vi "Read CellPart.vi"(8 "error in (no error)":errorcluster, 11 "TreeDoubleClickMsg in":refnum<class "TreeDoubleClickMsg.lvclass">) -> (0 "error out":errorcluster, 2 "CellPart":T1(ring), 3 "TreeDoubleClickMsg out":refnum<class "TreeDoubleClickMsg.lvclass">)   [LabVIEW 2019, in "ActorEvents.lvlib" / "TreeDoubleClickMsg.lvclass"]
uses:
  <vilib>/gpm_packages/@cs/mva-viewable/Source/ActorEvents/IEventAggregator Messages/TreeDoubleClickMsg/TreeDoubleClickMsg.lvclass
  <vilib>/gpm_packages/@cs/mva-viewable/Source/ActorEvents/IEventAggregator Messages/TreeDoubleClickMsg/TreeDoubleClickMsg.lvclass/TreeDoubleClickMsg.ctl
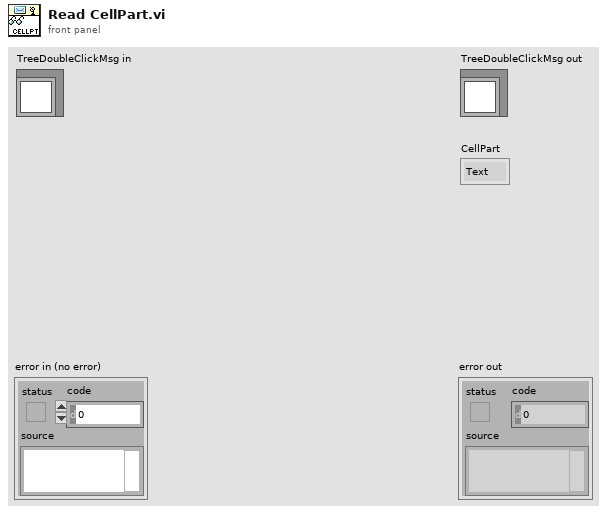
[diagram p1: front panel]
types:
  T1 = enum16{"Text", "Background", "Item Symbol", "Open/Close Symbol", "Hierarchy Lines", "Right Border", "Bottom Border", "Bottom Right Corner", "Unknown Part"}
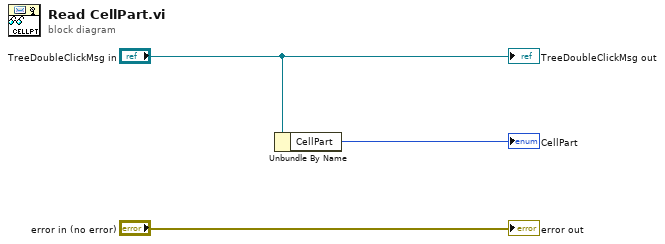
[diagram p0: block diagram]
diagram:
  n1 = Unbundle By Name("TreeDoubleClickMsg in") -> ("CellPart"=→"CellPart":T1)
  "error out" <- "error in (no error)"
  "TreeDoubleClickMsg out" <- "TreeDoubleClickMsg in"
